vi "Acquire_Path_Alias_Name.vi"(10 "Cluster of 7 Type Data":T2(array[cluster])) -> (0 "Path Coodinate Array":dbl[][](array[numeric]), 1 "All Path Array":string[](array[string]), 2 "Alias Array":string[](array[string]), 3 "District Name Array":string[](array[string]))   [LabVIEW 2014]
doc: "从簇数据中得到节点坐标数组"
uses:
  <vilib>/Analysis/Matrix/Datatypes/RealMatrix.ctl
  <vilib>/Analysis/Matrix/NI_Matrix.lvlib
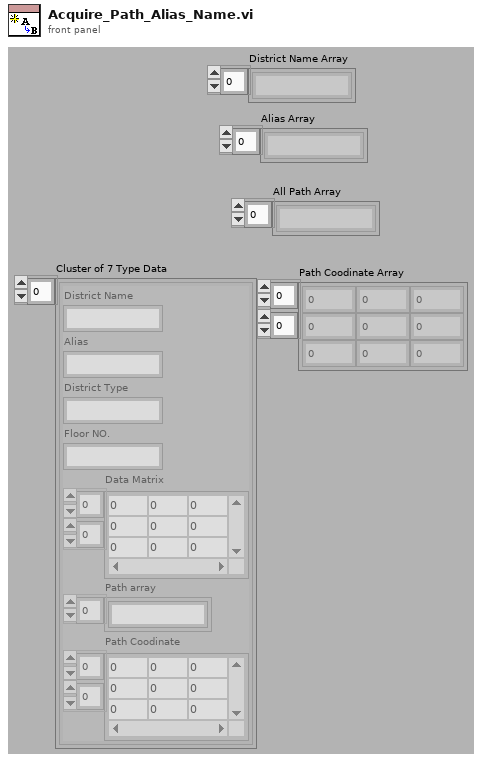
[diagram p1: front panel]
types:
  T1 = typedef "NI_Matrix.lvlib/RealMatrix.ctl" = dbl[][]
  T2 = cluster{"District Name":string, "Alias":string, "District Type":string, "Floor NO.":string, "Data Matrix":T1, "Path array":string[], "Path Coodinate":T1}[]
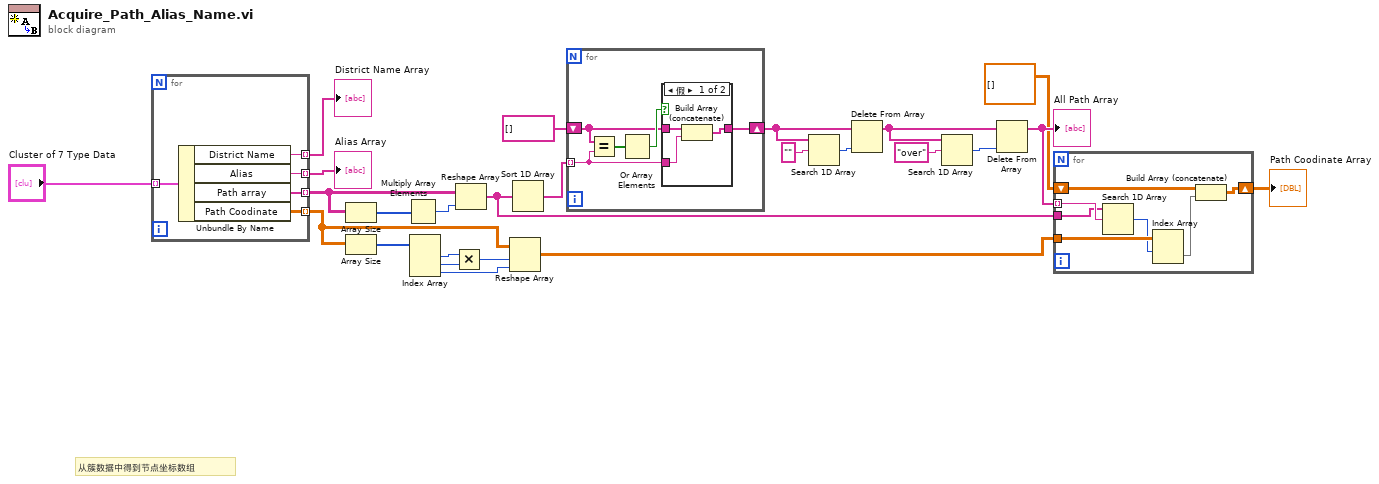
[diagram p0: block diagram]
diagram:
  # "从簇数据中得到节点坐标数组"
  n1 = for {
    tunnel: "Cluster of 7 Type Data" -> [w30] mode=indexing
    tunnel: [w28] -> w20 mode=indexing
    tunnel: [w29] -> w23 mode=indexing
    tunnel: [w27] -> w13 mode=indexing
    tunnel: [w26] -> w10 mode=indexing
    n2 = Unbundle By Name(w30) -> ("District Name"=w28:string, "Alias"=w27:string, "Path array"=w29:string[], "Path Coodinate"=w26:T1)
  }
  "District Name Array" <- w20
  "Alias Array" <- w13
  n3 = Array Size(array=w23) -> (size(s)=w25:i32[])
  n4 = Array Size(array=w10) -> (size(s)=w11:i32[])
  n5 = Multiply Array Elements(1:w25) -> (0:w24:i32)
  n6 = Index Array(array=w11) -> (element #1=w7:i32, element #2=w6:i32, element #3=w9:i32)  [unwired: 3 in]
  n7 = Multiply(x=w7, y=w6) -> (x*y=w8:i32)
  n8 = Reshape Array(w23, w24) -> (w4:string[])
  n9 = Reshape Array(w10, w8, w9) -> (w3:dbl[][])
  n10 = Sort 1D Array(array=w4) -> (sorted array=w22:string[])
  n11 = for {
    tunnel: w22 -> [w31] mode=indexing
    shift-right: [w32] -> w14
    shift-left: string[] [] -> [w33]
    n12 = Equal?(x=w33, y=w31) -> (x = y?=w35:bool[])
    n13 = Or Array Elements(Boolean array=w35) -> (logical OR=w34:bool)
    n14 = case shown="假" w34 {
      tunnel: w33 -> [w38 w39]
      tunnel: [w36 w39] -> w32
      tunnel: w31 -> [w37 _]
      frame False {
        n15 = Build Array (concatenate)(w38, w37) -> (w36:string[])
      }
      frame True {
      }
    }
  }
  n16 = Search 1D Array(1D array=w14, element="" ("元素")) -> (index of element=w18:i32)  [unwired: 1 in]
  n17 = Delete From Array(array=w14, index=w18) -> (array with subset deleted=w15:string[])  [unwired: 1 in, 1 out]
  n18 = Search 1D Array(1D array=w15, element="over" ("元素")) -> (index of element=w17:i32)  [unwired: 1 in]
  n19 = Delete From Array(array=w15, index=w17) -> (array with subset deleted=w5:string[])  [unwired: 1 in, 1 out]
  "All Path Array" <- w5
  n20 = for {
    tunnel: w5 -> [w46] mode=indexing
    tunnel: w4 -> [w45]
    tunnel: w3 -> [w44]
    shift-right: [w41] -> w1
    shift-left: dbl[][] [] -> [w40]
    n21 = Search 1D Array(1D array=w45, element=w46) -> (index of element=w43:i32)  [unwired: 1 in]
    n22 = Index Array(array=w44, index (row)=w43) -> (element=w42:dbl[])  [unwired: 1 in]
    n23 = Build Array (concatenate)(w40, w42) -> (w41:dbl[][])
  }
  "Path Coodinate Array" <- w1
